vi "QuickDropExamples.vi"(4 "String":string, 5 "Numeric":dbl format="%#_13g") -> (1 "Boolean":bool=TRUE)   [LabVIEW 2020]
panel:
  in  "Numeric 2":dbl format="%#_13g"
  in  "String 2":string
  out "Boolean 2":bool=TRUE
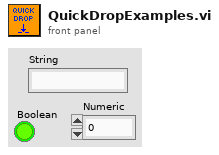
[diagram p1: front panel]
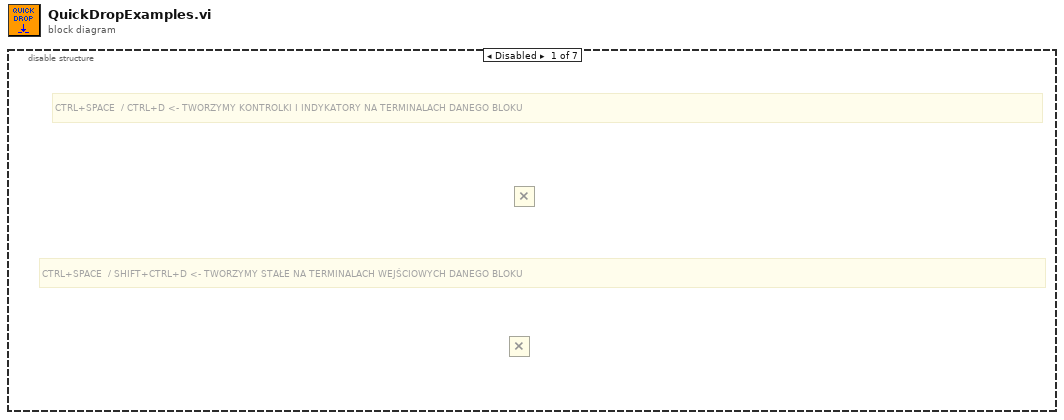
[diagram p0: block diagram]
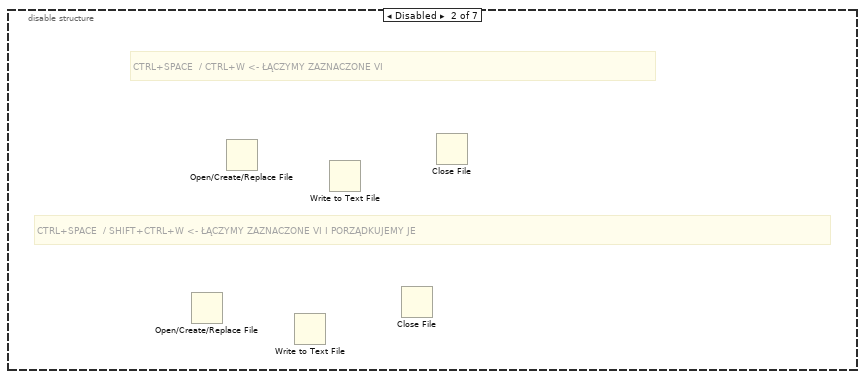
[diagram p2: hidden frame]
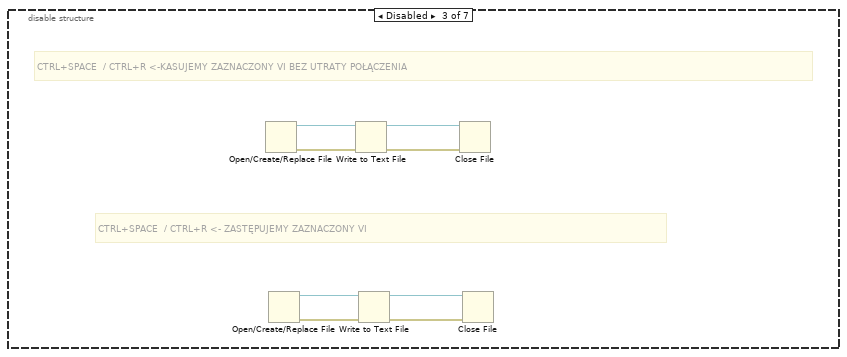
[diagram p3: hidden frame]
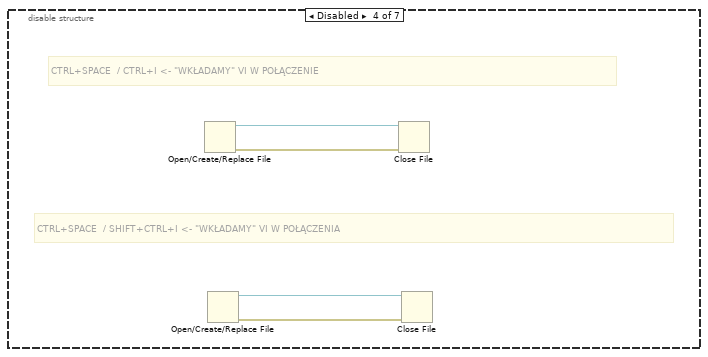
[diagram p4: hidden frame]
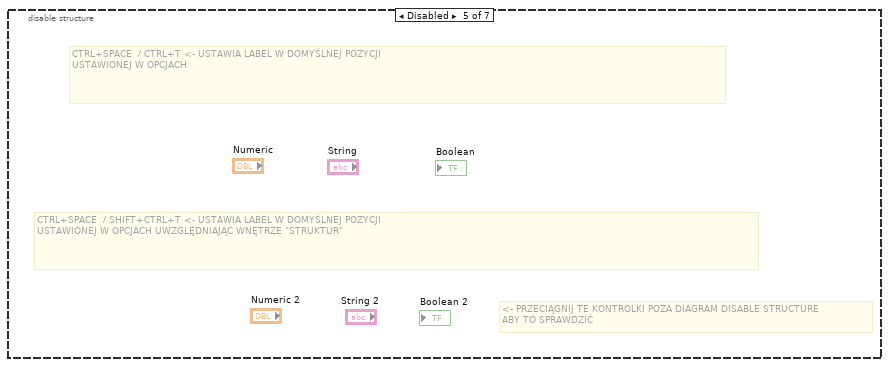
[diagram p5: hidden frame]
diagram:
  n1 = disable-structure shown="Disabled" {
    frame Disabled {
      # "CTRL+SPACE  / SHIFT+CTRL+D <- TWORZYMY STAŁE NA TERMINALACH WEJŚCIOWYCH DANEGO BLOKU"
      # "CTRL+SPACE  / CTRL+D <- TWORZYMY KONTROLKI I INDYKATORY NA TERMINALACH DANEGO BLOKU"
      n2 = Multiply() -> ()  [unwired: 2 in, 1 out]
      n3 = Multiply() -> ()  [unwired: 2 in, 1 out]
    }
    frame Disabled {
      # "CTRL+SPACE  / SHIFT+CTRL+W <- ŁĄCZYMY ZAZNACZONE VI I PORZĄDKUJEMY JE"
      # "CTRL+SPACE  / CTRL+W <- ŁĄCZYMY ZAZNACZONE VI"
      n4 = Open/Create/Replace File() -> ()  [unwired: 6 in, 3 out]
      n5 = Open/Create/Replace File() -> ()  [unwired: 6 in, 3 out]
      n6 = Write to Text File() -> ()  [unwired: 4 in, 3 out]
      n7 = Write to Text File() -> ()  [unwired: 4 in, 3 out]
      n8 = Close File() -> ()  [unwired: 2 in, 2 out]
      n9 = Close File() -> ()  [unwired: 2 in, 2 out]
    }
    frame Disabled {
      # "CTRL+SPACE  / CTRL+R <- ZASTĘPUJEMY ZAZNACZONY VI"
      # "CTRL+SPACE  / CTRL+R <-KASUJEMY ZAZNACZONY VI BEZ UTRATY POŁĄCZENIA"
      n10 = Open/Create/Replace File() -> (refnum out=w8:refnum<file>, error out=w7:errorcluster)  [unwired: 6 in, 1 out]
      n11 = Open/Create/Replace File() -> (refnum out=w1:refnum<file>, error out=w2:errorcluster)  [unwired: 6 in, 1 out]
      n12 = Write to Text File(file (use dialog)=w8, error in=w7) -> (refnum out=w6:refnum<file>, error out=w5:errorcluster)  [unwired: 2 in, 1 out]
      n13 = Write to Text File(file (use dialog)=w1, error in=w2) -> (refnum out=w3:refnum<file>, error out=w4:errorcluster)  [unwired: 2 in, 1 out]
      n14 = Close File(refnum=w6, error in=w5) -> ()  [unwired: 2 out]
      n15 = Close File(refnum=w3, error in=w4) -> ()  [unwired: 2 out]
    }
    frame Disabled {
      # "CTRL+SPACE  / SHIFT+CTRL+I <- \"WKŁADAMY\" VI W POŁĄCZENIA"
      # "CTRL+SPACE  / CTRL+I <- \"WKŁADAMY\" VI W POŁĄCZENIE"
      n16 = Open/Create/Replace File() -> (refnum out=w12:refnum<file>, error out=w11:errorcluster)  [unwired: 6 in, 1 out]
      n17 = Open/Create/Replace File() -> (refnum out=w9:refnum<file>, error out=w10:errorcluster)  [unwired: 6 in, 1 out]
      n18 = Close File(refnum=w12, error in=w11) -> ()  [unwired: 2 out]
      n19 = Close File(refnum=w9, error in=w10) -> ()  [unwired: 2 out]
    }
    frame Disabled {
      # "<- PRZECIĄGNIJ TE KONTROLKI POZA DIAGRAM DISABLE STRUCTURE\nABY TO SPRAWDZIĆ"
      # "CTRL+SPACE  / SHIFT+CTRL+T <- USTAWIA LABEL W DOMYŚLNEJ POZYCJI \nUSTAWIONEJ W OPCJACH UWZGLĘDNIAJĄC WNĘTRZE \"STRUKTUR\""
      # "CTRL+SPACE  / CTRL+T <- USTAWIA LABEL W DOMYŚLNEJ POZYCJI \nUSTAWIONEJ W OPCJACH"
    }
    frame Disabled {
      # "Przykład na block front panelu !"
      # "CTRL+SPACE  / CTRL+F <- USTAWIA KONTROLKI I INDYKATORY NA FRONT PANELU\nZGODNIE Z CONNECTOR PANE"
    }
    frame Enabled {
      # "CTRL+SPACE <- OKNO QUICK DROP"
    }
  }
